vi "16TVTI-ReadHeaterPercent.vi"(3 "ITC IO Info":T1={"Com Port"=1, "ISOBUS Address"=1, "GPIB Address"=1, "Communication"=enum."ISOBUS"}) -> (0 "Actual heater  %":dbl format="%.2f", 1 "ITC IO Info":T1={"Com Port"=1, "ISOBUS Address"=1, "GPIB Address"=1, "Communication"=enum."ISOBUS"})   [LabVIEW 2016]
doc: "Reads the heater output."
uses:
  Equipment/Oxford Software/Oxsoft/ITCSUBS.LLB/ITCIO.ctl
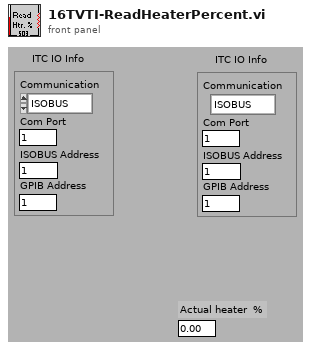
[diagram p1: front panel]
types:
  T1 = typedef "ITCIO.ctl" = cluster{"Com Port":i32, "ISOBUS Address":i32, "GPIB Address":i16, "Communication":enum16{"RS232", "ISOBUS", "GPIB", "Gateway"}}
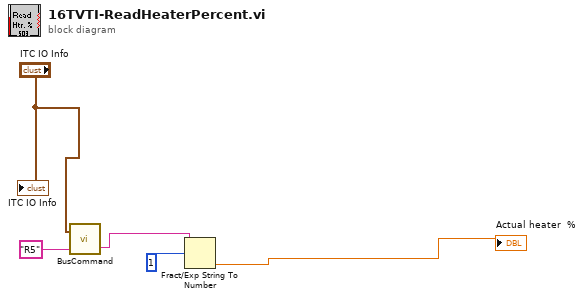
[diagram p0: block diagram]
diagram:
  n1 = call "BusCommand.vi"("Command"="R5", "Instrument address (in)"="ITC IO Info") -> ("Reply"=w4:string)  [unwired: 1 out]
  n2 = Fract/Exp String To Number(string=w4, offset=1) -> (number=→"Actual heater  %":dbl)  [unwired: 2 in, 1 out]
  "ITC IO Info" <- "ITC IO Info"
